vi "Save to Excel-12 (SubVI).vi"(0 "File Path Input":path, 1 "Change Save Location?":bool, 2 "Save (Enable/Signal)":bool, 3 "Save Interval (s)":dbl=1.0, 4 "Manual Save Interval?":bool, 5 "Error Input":errorcluster, 6 "File Configuration":T1={"Row Limit"=65500.0, "Title Block?"=TRUE, "Column Headers?"=TRUE, "Include Time & Elapsed Time?"=TRUE, "Default File Name"="Data", "Data Array Precision"=3, "Include Comments?"=TRUE, "New File Daily?"=TRUE}, 7 "Reset Elapsed Time":bool, 9 "Data Array (Row)":dbl[](array[numeric]), 11 "Title Block Text Array":string[](array[string]), 13 "Column Header Text Array":string[](array[string]), 19 "Comments":string) -> (14 "File Path Output":path, 15 "# of Rows Saved":dbl, 16 "Elapsed Time":string="00:00:00", 17 "Save Indicator":bool, 18 "Error Output":errorcluster)   [LabVIEW 2012]
uses:
  <vilib>/Utility/file.llb/Write To Spreadsheet File (string).vi
panel:
  out "Elapsed Time (s)":dbl
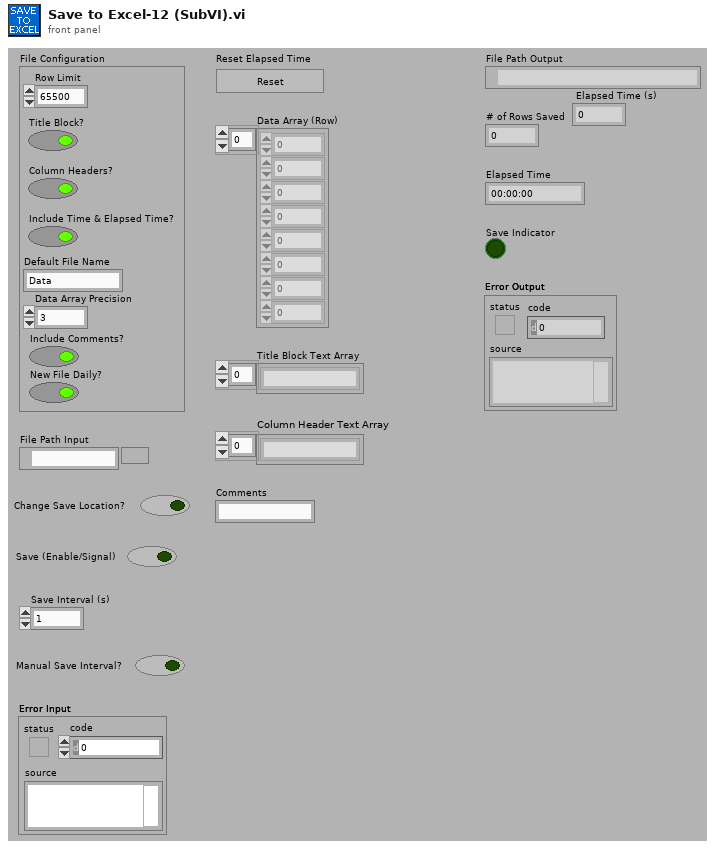
[diagram p1: front panel]
types:
  T1 = cluster{"Row Limit":dbl, "Title Block?":bool, "Column Headers?":bool, "Include Time & Elapsed Time?":bool, "Default File Name":string, "Data Array Precision":i16, "Include Comments?":bool, "New File Daily?":bool}
  T2 = typedef "LVDateTimeRec.ctl" = cluster{"fractional second":dbl, "second":i32, "minute":i32, "hour":i32, "day of month":i32, "month":i32, "year":i32, "day of week":i32, "day of year":i32, "DST":i32}
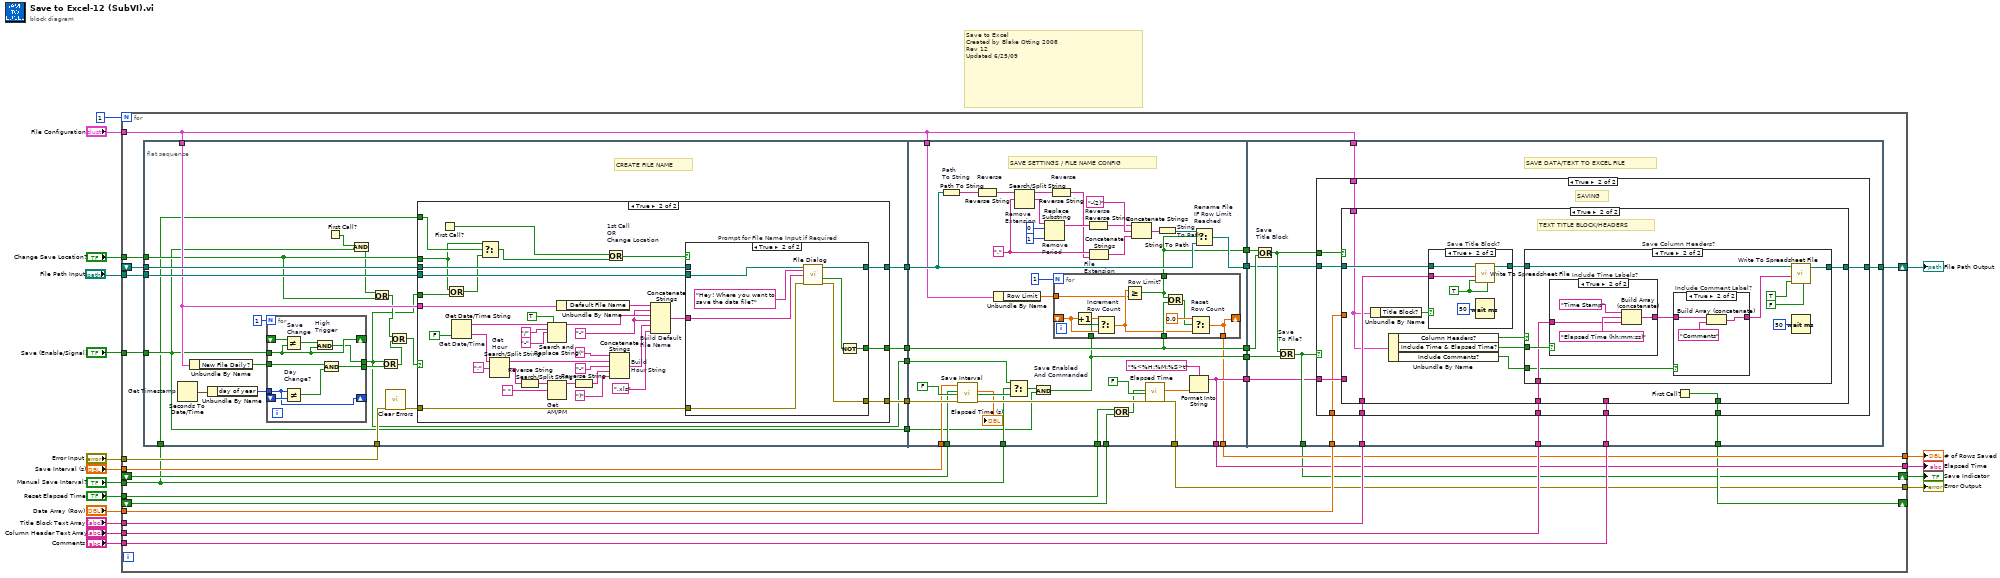
[diagram p0: block diagram]
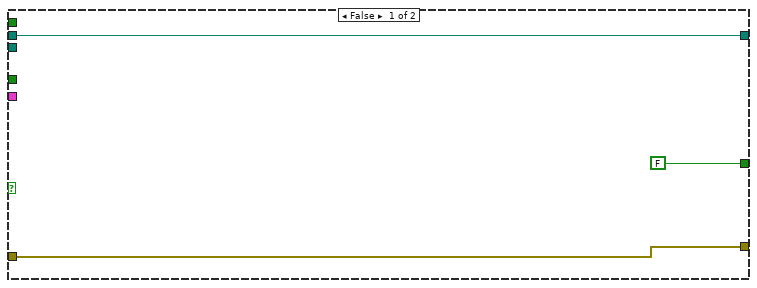
[diagram p2: hidden frame]
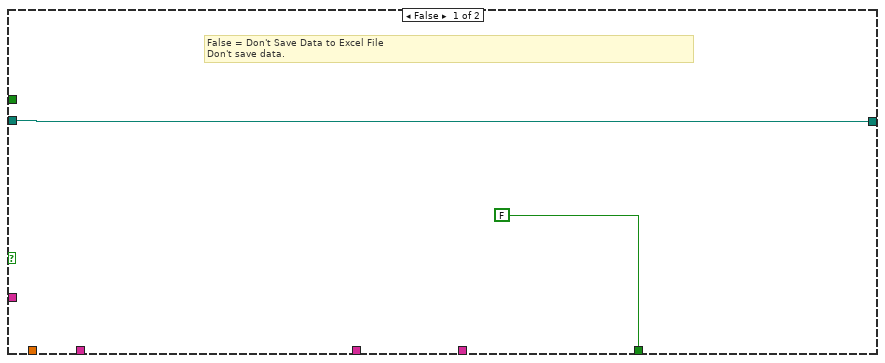
[diagram p4: hidden frame]
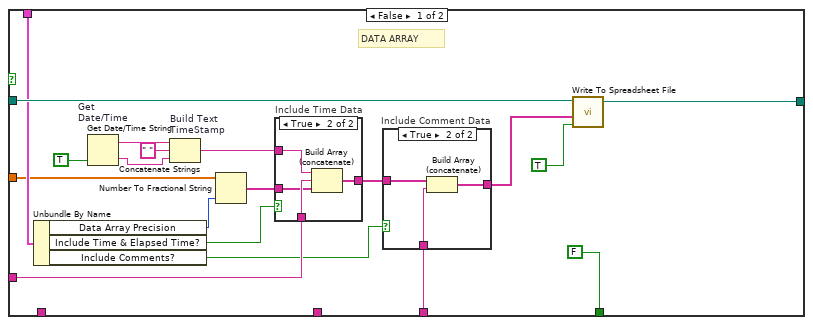
[diagram p5: hidden frame]
diagram:
  # "Save to Excel\nCreated by Blake Otting 2008\nRev 12 \nUpdated 6/25/09"
  n1 = for {
    N: 1 -> [_]
    tunnel: "File Path Input" -> [w33]
    tunnel: "Error Input" -> [w49]
    tunnel: "Change Save Location?" -> [w48]
    tunnel: "Save (Enable/Signal)" -> [w25]
    tunnel: "Data Array (Row)" -> [w36]
    tunnel: "Column Header Text Array" -> [w35]
    tunnel: "File Configuration" -> [w21]
    tunnel: "Reset Elapsed Time" -> [w22]
    shift-right: [w28] -> w16
    shift-left: _ -> [w44]
    tunnel: "Manual Save Interval?" -> [w20]
    tunnel: "Save Interval (s)" -> [w26]
    shift-right: [w29] -> _
    shift-left: _ -> [w23]
    tunnel: "Title Block Text Array" -> [w37]
    tunnel: "Comments" -> [w34]
    shift-right: [w38] -> w14
    shift-left: _ -> [w32]
    tunnel: [w30] -> w15
    tunnel: [w27] -> w17
    tunnel: [w31] -> w18
    n2 = flat-sequence {
      tunnel: w32 -> [w69]
      tunnel: w33 -> [w68]
      tunnel: w49 -> [w60]
      tunnel: w48 -> [w55]
      tunnel: w21 -> [w62]
      tunnel: [w71] -> w47
      tunnel: [w70] -> w46
      tunnel: [w67] -> w45
      tunnel: w25 -> [w52]
      tunnel: [w52] -> w24
      tunnel: w20 -> [w51]
      tunnel: [w50] -> w19
      tunnel: [w158] -> w43
      tunnel: [w155] -> w42
      tunnel: [w154] -> w41
      tunnel: [w146] -> w40
      tunnel: [w141] -> w39
      tunnel: [w150] -> w27
      tunnel: w21 -> [w156]
      tunnel: w44 -> [w143]
      tunnel: w20 -> [w144]
      tunnel: w45 -> [w157]
      tunnel: w46 -> [w147]
      tunnel: w47 -> [w155]
      tunnel: [w136] -> w31
      tunnel: [w141] -> w30
      tunnel: w26 -> [w140]
      tunnel: w24 -> [w139]
      tunnel: w23 -> [w135]
      tunnel: w22 -> [w134]
      tunnel: w19 -> [w131]
      tunnel: w43 -> [w192]
      tunnel: w42 -> [w195]
      tunnel: w41 -> [w196]
      tunnel: w40 -> [w193]
      tunnel: w39 -> [w185]
      tunnel: [w191] -> w38
      tunnel: w37 -> [w190]
      tunnel: w36 -> [w189]
      tunnel: w35 -> [w188]
      tunnel: w34 -> [w187]
      tunnel: [w186] -> w28
      tunnel: [w184] -> w29
      tunnel: w21 -> [w183]
      frame #0 {
        # "CREATE FILE NAME"
        n3 = Seconds To Date/Time "Get Timestamp"() -> (date time rec=w64:T2)  [unwired: 2 out]
        n4 = Unbundle By Name(w62) -> ("New File Daily?"=w66:bool)
        n5 = Unbundle By Name(w64) -> ("day of year"=w65:i32)
        n6 = for {
          N: 1 -> [_]
          tunnel: w52 -> [w78]
          shift-right: [w78] -> _
          shift-left: _ -> [w80]
          tunnel: [w77] -> w50
          tunnel: w65 -> [w75]
          shift-right: [w75] -> _
          shift-left: _ -> [w76]
          tunnel: w66 -> [w73]
          tunnel: [w72] -> w61
          n7 = Not Equal? "Save\nChange"(x=w80, y=w78) -> (x != y?=w79:bool)
          n8 = Not Equal? "Day\nChange?"(x=w75, y=w76) -> (x != y?=w74:bool)
          n9 = And "High\nTrigger"(x=w79, y=w78) -> (x .and. y?=w77:bool)
          n10 = And(x=w73, y=w74) -> (x .and. y?=w72:bool)
        }
        n11 = First Call?() -> (First Call?: T/F=w58:bool)
        n12 = And(x=w58, y=w52) -> (x .and. y?=w54:bool)
        n13 = Or(x=w54, y=w55) -> (x .or. y?=w53:bool)
        n14 = Or(x=w50, y=w61) -> (x .or. y?=w57:bool)
        n15 = call <vilib>:"Clear Errors.vi"("error in (no error)"=w60) -> ("error out"=w59:errorcluster)  [unwired: 6 out]
        n16 = Or(x=w53, y=w57) -> (x .or. y?=w56:bool)
        n17 = case shown="True" w56 {
          tunnel: [w83 w116] -> w67
          tunnel: w69 -> [w83 w89]
          tunnel: [FALSE ("First Call?: T/F") w118] -> w71
          tunnel: w68 -> [_ w117]
          tunnel: w55 -> [_ w86]
          tunnel: w59 -> [w81 w115]
          tunnel: [w81 w114] -> w70
          tunnel: w62 -> [_ w109]
          tunnel: w50 -> [_ w88]
          tunnel: w51 -> [_ w87]
          frame False {
          }
          frame True {
            w99 = "-" ("string")
            n18 = First Call?() -> (First Call?: T/F=w90:bool)
            n19 = Or(x=w86, y=w88) -> (x .or. y?=w85:bool)
            n20 = Get Date/Time String "Get Date/Time"(want seconds? (F)=FALSE) -> (date string=w93:string, time string=w92:string)  [unwired: 2 out]
            n21 = Select(t=w86, s=w87, f=w85) -> (s? t:f=w84:bool)
            n22 = Search/Split String "Get\nHour"(string=w92, search string/char (-)=":" ("search string")) -> (substring before match=w105:string, match + rest of string=w101:string)  [unwired: 2 out]
            n23 = Reverse String(1:w101) -> (0:w102:string)
            n24 = Search and Replace String(replace all?=TRUE ("replace all? (F)"), input string=w93, search string="/", replace string="-" ("replace string (\"\")")) -> (result string=w112:string)  [unwired: 1 in, 6 out]
            n25 = Search/Split String "Get\nAM/PM"(string=w102, search string/char (-)=" ") -> (substring before match=w104:string)  [unwired: 3 out]
            n26 = Unbundle By Name(w109) -> ("Default File Name"=w113:string)
            n27 = Reverse String(1:w104) -> (0:w106:string)
            n28 = Or "1st Call\nOR\nChange Location"(x=w90, y=w84) -> (x .or. y?=w119:bool)
            n29 = Concatenate Strings "Build\nHour String"("(" ("string"), w105, "-" ("search string/char (-)"), w106, ")" ("string")) -> (w95:string)
            n30 = Concatenate Strings "Build Default\nFile Name"(w113, w99, w112, w99, w95, ".xls" ("string")) -> (w108:string)
            n31 = case "Prompt for File Name Input if Required" shown="True" w119 {
              selector: w119 -> [w121 _]
              tunnel: [w121 w129] -> w118
              tunnel: w117 -> [_ w128]
              tunnel: [w122 w127] -> w116
              tunnel: w89 -> [w122 _]
              tunnel: w115 -> [w120 w123]
              tunnel: [w120 w125] -> w114
              tunnel: w108 -> [_ w124]
              frame False {
              }
              frame True {
                n32 = call "File Dialog"("start path"=w128, "prompt"="Hey! Where you want to save the data file?", "default name"=w124, "error in"=w123) -> ("selected path"=w127:path, "cancelled"=w130:bool, "error out"=w125:errorcluster)  [unwired: 3 in, 6 out]
                n33 = Not(x=w130) -> (.not. x?=w129:bool)
              }
            }
          }
        }
      }
      frame #1 {
        w168 = "." ("search string/char (-)")
        # "SAVE SETTINGS / FILE NAME CONFIG"
        n34 = Path To String "Path\nTo String"(path=w157) -> (string=w160:string)
        n35 = call "Save Interval"("Time Target (s)"=w140, "Reset"=w143, "Auto Reset"=FALSE, "error in (no error)"=w147) -> ("Elapsed Time (s)"=→"Elapsed Time (s)":dbl, "Time has Elapsed"=w145:bool, "error out"=w149:errorcluster)  [unwired: 1 in, 12 out]
        n36 = Reverse String "Reverse"(1:w160) -> (0:w161:string)
        n37 = Unbundle By Name(w156) -> ("Row Limit"=w138:dbl)
        n38 = Select(t=w131, s=w144, f=w145) -> (s? t:f=w142:bool)
        n39 = Search/Split String "Remove\nExtension"(string=w161, search string/char (-)=w168) -> (substring before match=w162:string, match + rest of string=w164:string)  [unwired: 2 out]
        n40 = And "Save Enabled\nAnd Commanded"(x=w142, y=w139) -> (x .and. y?=w146:bool)
        n41 = Replace Substring "Remove\nPeriod"(2:1 ("length (len. of substring)"), 3:0 ("offset (0)"), 5:w164) -> (1:w165:string)  [unwired: 2 out]
        n42 = Reverse String "Reverse"(1:w162) -> (0:w163:string)
        n43 = for {
          N: 1 -> [_]
          tunnel: w155 -> [w178]
          tunnel: [w176] -> w154
          tunnel: w146 -> [w177]
          shift-right: [w173] -> _
          shift-left: _ -> [w180]
          tunnel: w138 -> [w174]
          tunnel: [w173] -> w136
          n44 = Increment(x=w180) -> (x+1=w182:dbl)
          n45 = Select "Increment\nRow Count"(t=w182, s=w177, f=w180) -> (s? t:f=w175:dbl)
          n46 = Greater Or Equal? "Row Limit?"(x=w175, y=w174) -> (x >= y?=w176:bool)
          n47 = Or(x=w176, y=w178) -> (x .or. y?=w179:bool)
          n48 = Select "Reset\nRow Count"(t=0.0, s=w179, f=w175) -> (s? t:f=w173:dbl)
        }
        n49 = Reverse String "Reverse"(1:w165) -> (0:w169:string)
        n50 = Concatenate Strings "File\nExtension"(w168, w163) -> (w159:string)
        n51 = Or(x=w134, y=w135) -> (x .or. y?=w133:bool)
        n52 = Concatenate Strings(w169, "-(2)", w159) -> (w170:string)
        n53 = call "Elapsed Time"("Reset"=w133, "Auto Reset"=FALSE, "error in (no error)"=w149) -> ("Elapsed Time (s)"=w152:dbl, "error out"=w150:errorcluster)  [unwired: 2 in, 13 out]
        n54 = String To Path "String\nTo Path"(string=w170) -> (path=w171:path)
        n55 = Format Into String(format string="%<%H:%M:%S>t", w152) -> (resulting string=w141:string)  [unwired: 2 in, 1 out]
        n56 = Select "Rename File\nIF Row Limit\nReached"(t=w171, s=w154, f=w157) -> (s? t:f=w158:path)
      }
      frame #2 {
        # "SAVE DATA/TEXT TO EXCEL FILE"
        n57 = Or "Save\nTitle Block"(x=w196, y=w195) -> (x .or. y?=w194:bool)
        n58 = Or "Save\nTo File?"(x=w194, y=w193) -> (x .or. y?=w186:bool)
        n59 = case shown="True" w186 {
          tunnel: [w198 w208] -> w191
          tunnel: w192 -> [w198 w207]
          tunnel: w194 -> [_ w206]
          tunnel: [FALSE ("First Call?: T/F") w205] -> w184
          tunnel: w183 -> [_ w204]
          tunnel: w185 -> [_ w203]
          tunnel: w190 -> [_ w200]
          tunnel: w189 -> [_ w202]
          tunnel: w188 -> [_ w201]
          tunnel: w187 -> [_ w199]
          frame False {
            # "False = Don't Save Data to Excel File\nDon't save data."
          }
          frame True {
            # "SAVING"
            n60 = case shown="True" w206 {
              tunnel: [w227 w245] -> w208
              tunnel: w207 -> [w225 w247]
              tunnel: w200 -> [_ w239]
              tunnel: w201 -> [_ w244]
              tunnel: w203 -> [w223 _]
              tunnel: [FALSE ("First Call?: T/F") w243] -> w205
              tunnel: w199 -> [w219 _]
              tunnel: w204 -> [w215 w238]
              tunnel: w202 -> [w209 _]
              frame False {
                # "DATA ARRAY"
                n61 = Unbundle By Name(w215) -> ("Data Array Precision"=w218:i16, "Include Time & Elapsed Time?"=w217:bool, "Include Comments?"=w216:bool)
                n62 = Get Date/Time String "Get \nDate/Time"(want seconds? (F)=TRUE) -> (date string=w214:string, time string=w211:string)  [unwired: 2 out]
                n63 = Concatenate Strings "Build Text\nTimeStamp"(w214, " " ("string"), w211) -> (w210:string)
                n64 = Number To Fractional String(number=w209, precision (6)=w218) -> (F-format string=w224:string[])  [unwired: 2 out]
                n65 = case "Include Time Data" shown="True" w217 {
                  tunnel: w224 -> [w232 w233]
                  tunnel: w210 -> [_ w234]
                  tunnel: [w232 w236] -> w220
                  tunnel: w223 -> [_ w235]
                  frame False {
                  }
                  frame True {
                    n66 = Build Array (concatenate)(w234, w235, w233) -> (w236:string[])
                  }
                }
                n67 = case "Include Comment Data" shown="True" w216 {
                  tunnel: w219 -> [_ w231]
                  tunnel: [w228 w230] -> w221
                  tunnel: w220 -> [w228 w229]
                  frame False {
                  }
                  frame True {
                    n68 = Build Array (concatenate)(w229, w231) -> (w230:string[])
                  }
                }
                n69 = call-poly <vilib>:"Write To Spreadsheet File.vi"("append to file? (new file:F)"=TRUE, "1D data"=w221, "file path (dialog if empty)"=w225) -> ("new file path (Not A Path if cancelled)"=w227:path)  [unwired: 3 in, 2 out]
              }
              frame True {
                # "TEXT TITLE BLOCK/HEADERS"
                n70 = Unbundle By Name(w238) -> ("Title Block?"=w237:bool)
                n71 = Unbundle By Name(w238) -> ("Column Headers?"=w242:bool, "Include Time & Elapsed Time?"=w241:bool, "Include Comments?"=w240:bool)
                n72 = case "Save Title Block?" shown="True" w237 {
                  tunnel: w247 -> [w268 w272]
                  tunnel: [w268 w271] -> w246
                  tunnel: w239 -> [_ w269]
                  frame False {
                  }
                  frame True {
                    w273 = TRUE ("transpose? (no:F)")
                    n73 = call-poly <vilib>:"Write To Spreadsheet File.vi"("transpose? (no:F)"=w273, "append to file? (new file:F)"=w273, "1D data"=w269, "file path (dialog if empty)"=w272) -> ("new file path (Not A Path if cancelled)"=w271:path)  [unwired: 2 in, 2 out]
                    n74 = Wait (ms)(milliseconds to wait=u32 50) -> ()  [unwired: 1 out]
                  }
                }
                n75 = case "Save Column Headers?" shown="True" w242 {
                  tunnel: w246 -> [w248 w254]
                  tunnel: [w248 w256] -> w245
                  tunnel: w244 -> [_ w252]
                  tunnel: w241 -> [_ w253]
                  tunnel: w240 -> [_ w249]
                  frame False {
                  }
                  frame True {
                    n76 = case "Include Time Labels?" shown="True" w253 {
                      tunnel: w252 -> [w263 w265]
                      tunnel: [w263 w264] -> w251
                      frame False {
                      }
                      frame True {
                        n77 = Build Array (concatenate)("Time Stamp", "Elapsed Time (hh:mm:ss)", w265) -> (w264:string[])
                      }
                    }
                    n78 = case "Include Comment Label?" shown="True" w249 {
                      tunnel: w251 -> [w259 w262]
                      tunnel: [w259 w260] -> w250
                      frame False {
                      }
                      frame True {
                        n79 = Build Array (concatenate)(w262, "Comments") -> (w260:string[])
                      }
                    }
                    n80 = call-poly <vilib>:"Write To Spreadsheet File.vi"("transpose? (no:F)"=FALSE, "append to file? (new file:F)"=TRUE ("transpose? (no:F)"), "1D data"=w250, "file path (dialog if empty)"=w254) -> ("new file path (Not A Path if cancelled)"=w256:path)  [unwired: 2 in, 2 out]
                    n81 = Wait (ms)(milliseconds to wait=u32 50) -> ()  [unwired: 1 out]
                  }
                }
                n82 = First Call?() -> (First Call?: T/F=w243:bool)
              }
            }
          }
        }
      }
    }
  }
  "# of Rows Saved" <- w18
  "Save Indicator" <- w16
  "File Path Output" <- w14
  "Error Output" <- w17
  "Elapsed Time" <- w15
